vi "setID.vi"(8 "error in (no error)":errorcluster, 10 "ID":u32, 11 "LLSearch in":refnum<class "LLSearch.lvclass">) -> (0 "error out":errorcluster, 3 "LLSearch out":refnum<class "LLSearch.lvclass">)   [LabVIEW 2009, in "LLSearch.lvclass"]
uses:
  LLSearch.lvclass
  LLSearch.lvclass/LLSearch.ctl
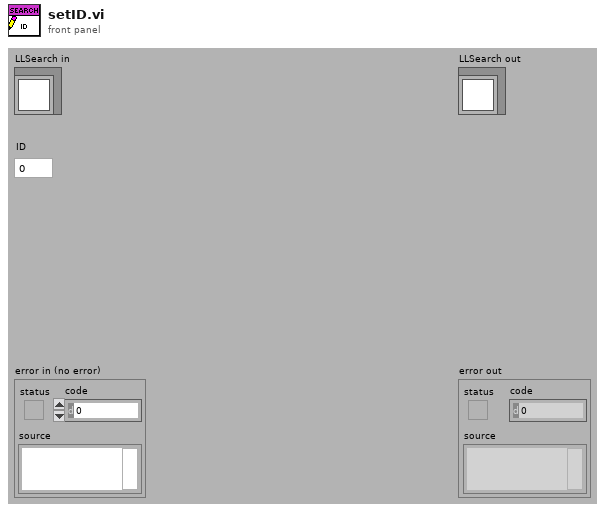
[diagram p1: front panel]
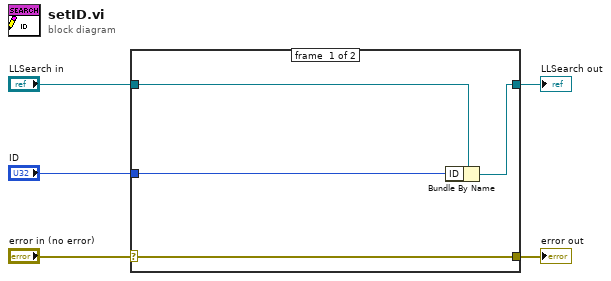
[diagram p0: block diagram]
diagram:
  n1 = case shown="No Error" "error in (no error)" {
    selector: "error in (no error)" -> [w9 w10]
    tunnel: [w9 w10] -> w4
    tunnel: [w7 w11] -> w2
    tunnel: "LLSearch in" -> [w8 w11]
    tunnel: "ID" -> [w6 _]
    frame #0 {
      n2 = Bundle By Name(cluster=w8, "ID"=w6) -> (w7:refnum<class "LLSearch.lvclass">)
    }
    frame #1 {
    }
  }
  "error out" <- w4
  "LLSearch out" <- w2
